vi "PathPlanner_GridPosition_CompareTo.vi"(9 "Other GridPosition":T1, 11 "GridPosition":T1) -> ()   [LabVIEW 2019, in "PathPlanner24.lvlib"]
uses:
  PathPlanner24.lvlib
  TypeDef/PathPlannerFinderGridPosition.ctl
panel:
  out "Compare":i32
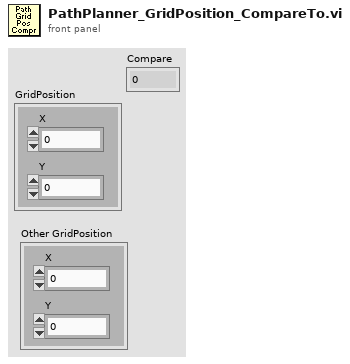
[diagram p1: front panel]
types:
  T1 = typedef "PathPlanner24.lvlib/PathPlannerFinderGridPosition.ctl" = cluster{"X":i32, "Y":i32}
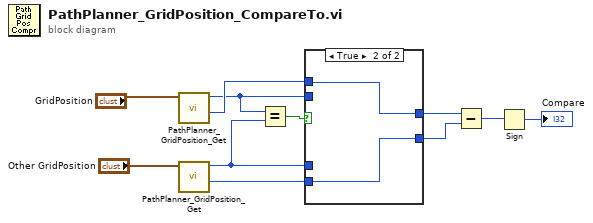
[diagram p0: block diagram]
diagram:
  n1 = call "PathPlanner_GridPosition_Get.vi"("GridPosition"="GridPosition") -> ("Int Y"=w8:i32, "Int X"=w2:i32)  [unwired: 9 in]
  n2 = call "PathPlanner_GridPosition_Get.vi"("GridPosition"="Other GridPosition") -> ("Int Y"=w7:i32, "Int X"=w1:i32)  [unwired: 9 in]
  n3 = Equal?(x=w2, y=w1) -> (x = y?=w9:bool)
  n4 = case shown="True" w9 {
    tunnel: w8 -> [_ w15]
    tunnel: w7 -> [_ w14]
    tunnel: [w13 w15] -> w6
    tunnel: [w12 w14] -> w5
    tunnel: w2 -> [w13 _]
    tunnel: w1 -> [w12 _]
    frame False {
    }
    frame True {
    }
  }
  n5 = Subtract(x=w6, y=w5) -> (x-y=w4:i32)
  n6 = Sign(1:w4) -> (0:→"Compare":i32)
